vi "GetWaveformData.vi"(8 "error in (no error)":errorcluster, 9 "Number of Samples":i32, 10 "Current Channel":string, 11 "Data Value Reference in":T3) -> (0 "error out":errorcluster, 3 "DataSet":T1)   [LabVIEW 2017, in "McsaTestPanel.lvlib"]
uses:
  <vilib>/addons/InsightCM/Devices/Shared/Mcsa/McsaTestPanel/McsaTestPanel.lvlib
  <vilib>/addons/InsightCM/Utilities/DataAccessors/controls/wfmSGL_DVR.ctl
  <vilib>/addons/InsightCM/MessageBus/Base/controls/DataSetByteData.ctl
  <vilib>/addons/InsightCM/MessageBus/Base/controls/KeyValuePair.ctl
  <vilib>/addons/InsightCM/Utilities/ChannelStatus/ChannelStatus.lvlib
  <vilib>/addons/InsightCM/Utilities/PropertyHelpers/PropertyHelpers.lvlib
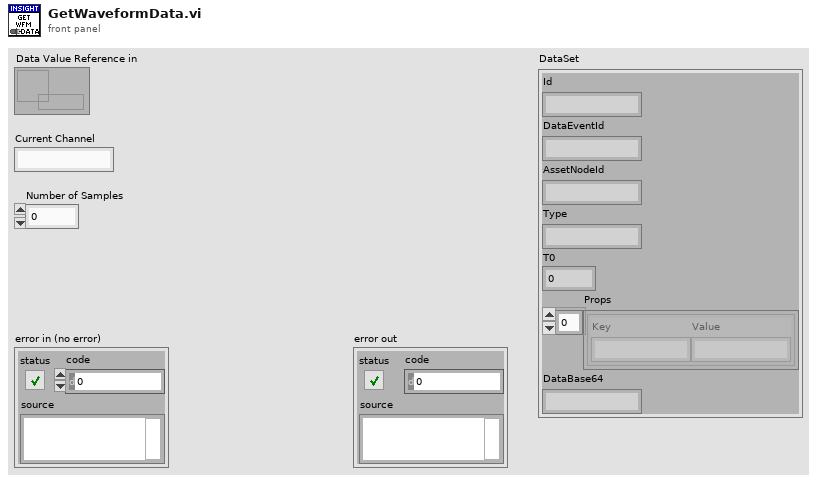
[diagram p1: front panel]
types:
  T1 = typedef "DataSetByteData.ctl" = cluster{"Id":string, "DataEventId":string, "AssetNodeId":string, "Type":string, "T0":i64, "Props":T2[], "DataBase64":string}
  T2 = typedef "KeyValuePair.ctl" = cluster{"Key":string, "Value":string}
  T3 = typedef "wfmSGL_DVR.ctl" = refnum<data-value>
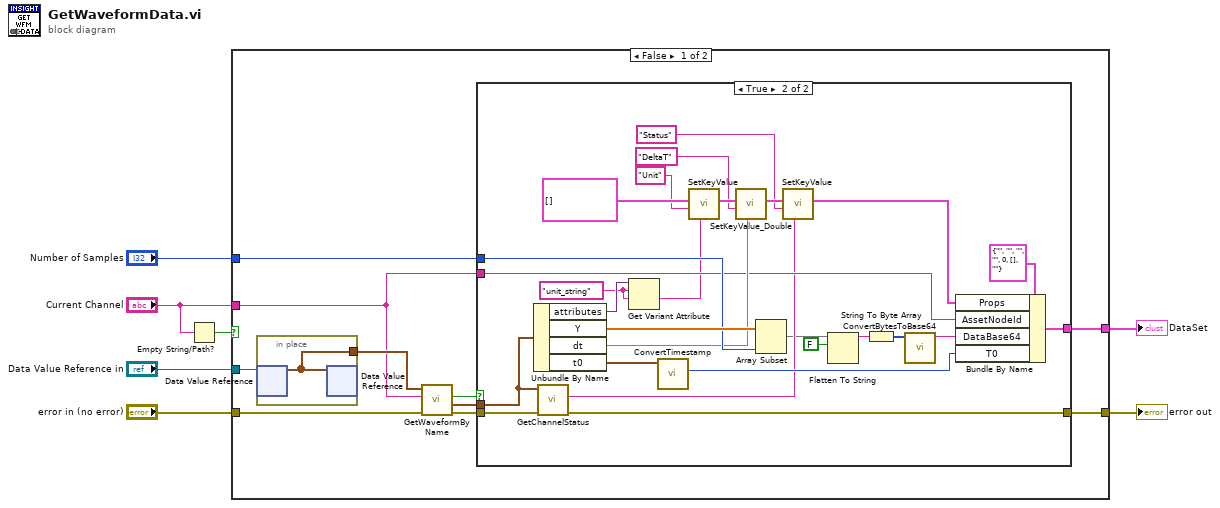
[diagram p0: block diagram]
diagram:
  n1 = Empty String/Path?(string/path="Current Channel") -> (empty?=w5:bool)
  n2 = case shown="False" w5 {
    tunnel: "Data Value Reference in" -> [w17 _]
    tunnel: [w13 w47] -> w3
    tunnel: "error in (no error)" -> [w16 w47]
    tunnel: "Current Channel" -> [w10 _]
    tunnel: "Number of Samples" -> [w9 _]
    tunnel: [w8 _] -> w1
    frame False {
      n3 = in-place {
        in-place-border: [w46] -> w15
        n4 = in-place-dvr #1(w17) -> (w46:waveform(sgl)[])  [unwired: 1 out]
        n5 = in-place-dvr #1(w46) -> ()  [unwired: 2 out]
      }
      n6 = call <vilib>:"GetWaveformByName.vi"("error in (no error)"=w16, "Channel Name"=w10, "Acq Waveforms"=w15) -> ("error out"=w12:errorcluster, "Waveform"=w11:waveform(sgl), "Found?"=w14:bool)  [unwired: 5 in, 1 out]
      n7 = case shown="True" w14 {
        tunnel: [w18 w44] -> w13
        tunnel: w12 -> [w18 w45]
        tunnel: w11 -> [_ w39]
        tunnel: w10 -> [_ w27]
        tunnel: w9 -> [_ w37]
        tunnel: [_ w42] -> w8
        frame False {
        }
        frame True {
          w40 = "unit_string" ("name")
          n8 = Unbundle By Name(w39) -> ("attributes"=w41:variant, "Y"=w38:sgl[], "dt"=w29:dbl, "t0"=w43:timestamp)
          n9 = call <vilib>:"GetChannelStatus.vi"("error in (no error)"=w45, "waveform in"=w39) -> ("error out"=w44:errorcluster, "channel status"=w26:string)  [unwired: 6 in, 2 out]
          n10 = Get Variant Attribute(Variant=w41, name=w40, default value (empty Variant)=w40) -> (value=w24:string)  [unwired: 1 in, 3 out]
          n11 = call <vilib>:"ConvertTimestamp.vi"("Time Stamp"=w43) -> ("Timestamp out"=w28:i64)  [unwired: 10 in]
          n12 = call <vilib>:"SetKeyValue.vi"("value"=w24, "key"="Unit", "key value pairs"=T2[] []) -> ("key value pairs out"=w35:T2[])  [unwired: 8 in]
          n13 = call <vilib>:"SetKeyValue_Double.vi"("value"=w29, "key"="DeltaT", "key value pairs"=w35) -> ("key value pairs out"=w36:T2[])  [unwired: 8 in]
          n14 = Array Subset(array=w38, length=w37) -> (w19:sgl[])  [unwired: 1 in]
          n15 = call <vilib>:"SetKeyValue.vi"("value"=w26, "key"="Status", "key value pairs"=w36) -> ("key value pairs out"=w33:T2[])  [unwired: 8 in]
          n16 = Flatten To String(anything=w19, prepend array or string size? (T)=FALSE) -> (data string=w23:string)  [unwired: 2 in, 2 out]
          n17 = String To Byte Array(string=w23) -> (unsigned byte array=w21:u8[])
          n18 = call <vilib>:"ConvertBytesToBase64.vi"("U8 array"=w21) -> ("base64 encoded"=w20:string)  [unwired: 10 in]
          n19 = Bundle By Name(cluster=T1 {"Id"="", "DataEventId"="", "AssetNodeId"="", "Type"="", "T0"=0, "Props"=[], "DataBase64"=""} ("DataSet"), "Props"=w33, "AssetNodeId"=w27, "DataBase64"=w20, "T0"=w28) -> (w42:T1)
        }
      }
    }
    frame True {
    }
  }
  "error out" <- w3
  "DataSet" <- w1
